vi "trigger.vi"(4 "In":waveform(dbl)) -> (1 "Out":waveform(dbl))   [LabVIEW 2012]
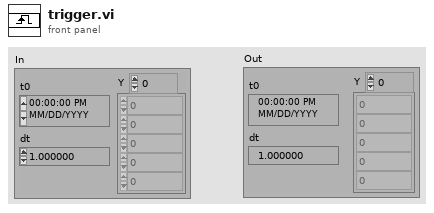
[diagram p1: front panel]
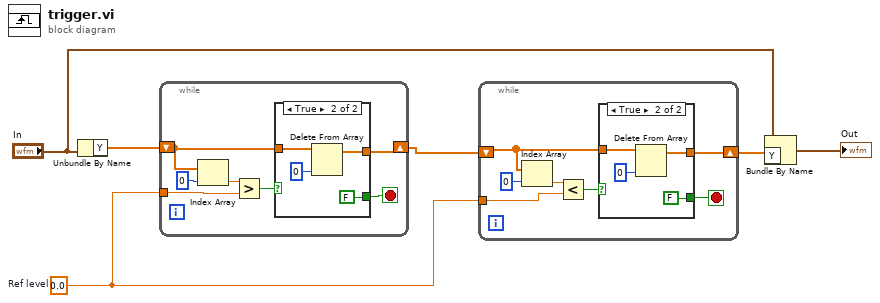
[diagram p0: block diagram]
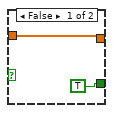
[diagram p2: hidden frame]
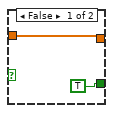
[diagram p3: hidden frame]
diagram:
  w4 = 0.0  # Ref level
  n1 = Unbundle By Name("In") -> ("Y"=w2:dbl[])
  n2 = while {
    shift-right: [w7] -> w3
    shift-left: w2 -> [w9]
    tunnel: w4 -> [w12]
    stop <- w10 stop-if-true
    n3 = Index Array(array=w9, index=0) -> (element=w13:dbl)
    n4 = Greater?(x=w13, y=w12) -> (0:w11:bool)
    n5 = case shown="True" w11 {
      tunnel: [TRUE FALSE] -> w10
      tunnel: w9 -> [w15 w18]
      tunnel: [w15 w16] -> w7
      frame False {
      }
      frame True {
        n6 = Delete From Array(array=w18, index=0) -> (array with subset deleted=w16:dbl[])  [unwired: 1 in, 1 out]
      }
    }
  }
  n7 = while {
    shift-right: [w22] -> w5
    shift-left: w3 -> [w23]
    tunnel: w4 -> [w20]
    stop <- w24 stop-if-true
    n8 = Index Array(array=w23, index=0) -> (element=w25:dbl)
    n9 = Less?(x=w25, y=w20) -> (x < y?=w26:bool)
    n10 = case shown="True" w26 {
      tunnel: [TRUE FALSE] -> w24
      tunnel: w23 -> [w28 w31]
      tunnel: [w28 w29] -> w22
      frame False {
      }
      frame True {
        n11 = Delete From Array(array=w31, index=0) -> (array with subset deleted=w29:dbl[])  [unwired: 1 in, 1 out]
      }
    }
  }
  n12 = Bundle By Name(cluster="In", "Y"=w5) -> (→"Out":waveform(dbl))
